vi "Run RT VI in project.vi"(5 "project target":string, 6 "configuration file path":path, 7 "ip address":string, 8 "error in (no error)":errorcluster, 9 "target alias":string, 10 "vi name":string, 11 "Project Path":path) -> (0 "error out":errorcluster, 1 "invoked VI error out":errorcluster, 2 "pass":bool, 3 "engine status":string)   [LabVIEW 2014]
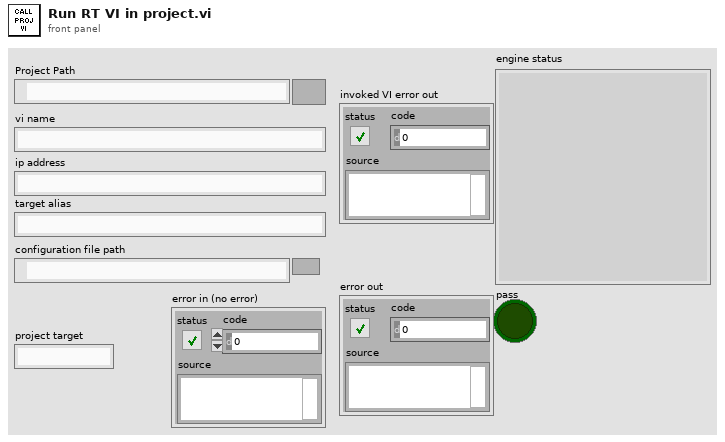
[diagram p1: front panel]
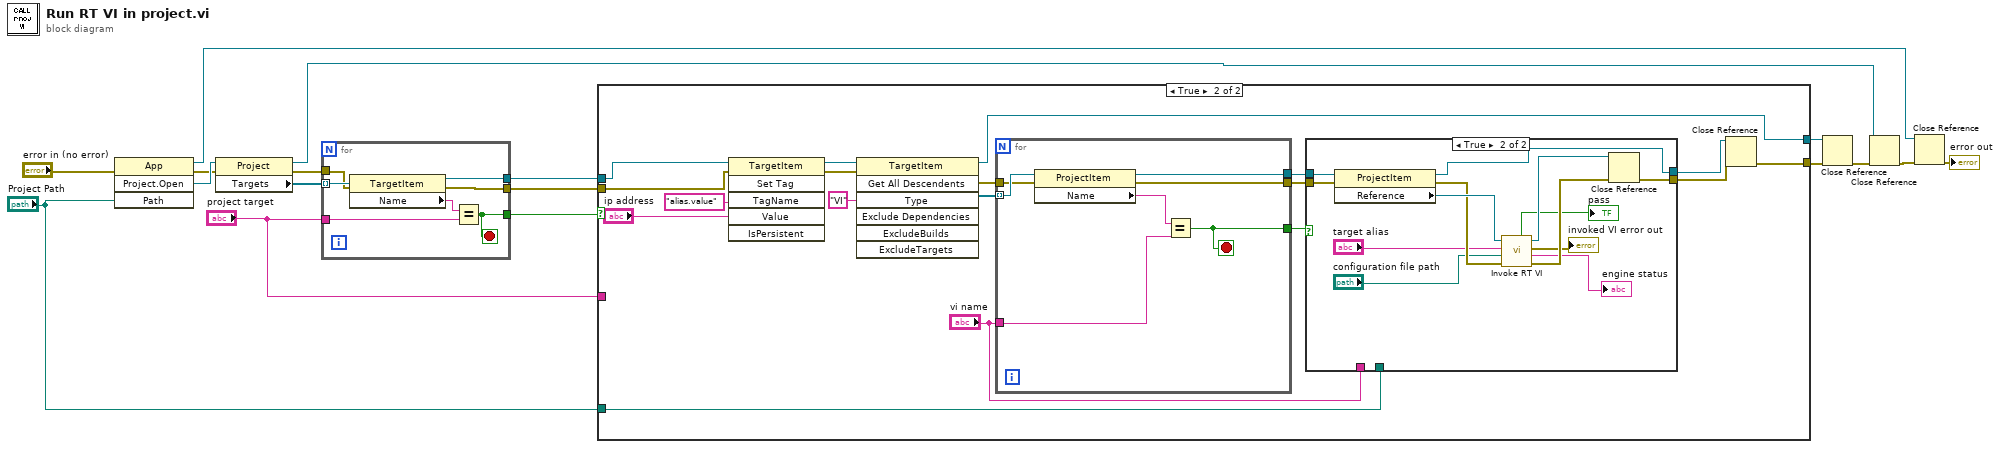
[diagram p0: block diagram]
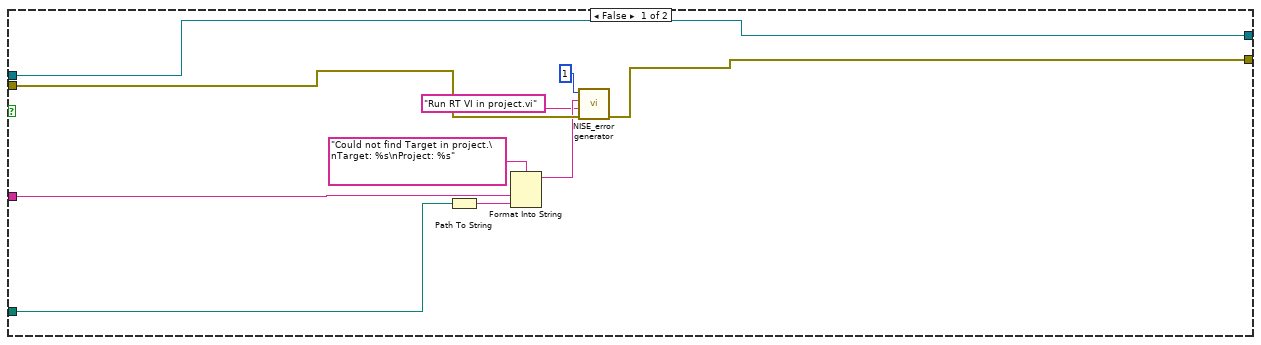
[diagram p2: hidden frame]
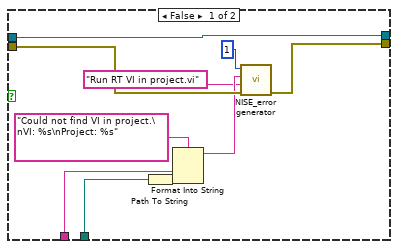
[diagram p3: hidden frame]
diagram:
  n1 = invoke class="App" method="Project.Open"(error in="error in (no error)", "Path"="Project Path") -> (reference out=w12:refnum<vi>, error out=w16:errorcluster, "Project:Open"=w17:refnum<vi>)  [unwired: 2 in, 1 out]
  n2 = property class="Project"(reference=w17, error in=w16) -> (reference out=w14:refnum<vi>, error out=w7:errorcluster, "Targets"=w15:refnum<vi>[])
  n3 = for {
    tunnel: w15 -> [w24] mode=indexing
    tunnel: [w23] -> w9
    tunnel: w7 -> [w21]
    tunnel: [w20] -> w6
    tunnel: [w19] -> w5
    tunnel: "project target" -> [w18]
    stop <- w19 stop-if-true
    n4 = property class="TargetItem"(reference=w24, error in=w21) -> (reference out=w23:refnum<vi>, error out=w20:errorcluster, "Name"=w22:string)
    n5 = Equal?(x=w22, y=w18) -> (x = y?=w19:bool)
  }
  n6 = case shown="True" w5 {
    tunnel: [w25 w35] -> w3
    tunnel: w9 -> [w34 w45]
    tunnel: "Project Path" -> [w33 w38]
    tunnel: w6 -> [w31 w37]
    tunnel: [w34 w36] -> w4
    tunnel: "project target" -> [w32 _]
    frame False {
      n7 = Path To String(path=w33) -> (string=w28:string)
      n8 = Format Into String(format string="Could not find Target in project.\nTarget: %s\nProject: %s" ("append error message"), w32, w28) -> (resulting string=w27:string)  [unwired: 2 in, 1 out]
      n9 = call <vilib>:"NISE_error generator.vi"("error in"=w31, "source"="Run RT VI in project.vi", "append error message"=w27, "error code (0)"=1) -> ("error out"=w25:errorcluster)  [unwired: 5 in]
    }
    frame True {
      n10 = invoke class="TargetItem" method="Set Tag"(reference=w45, error in=w37, "TagName"="alias.value" ("Tag Name"), "Value"="ip address") -> (reference out=w41:refnum<vi>, error out=w42:errorcluster)  [unwired: 2 in, 4 out]
      n11 = invoke class="TargetItem" method="Get All Descendents"(reference=w41, error in=w42, "Type"="VI") -> (reference out=w36:refnum<vi>, error out=w51:errorcluster, "All Descendents"=w52:refnum<vi>[])  [unwired: 4 in, 4 out]
      n12 = for {
        tunnel: w52 -> [w82] mode=indexing
        tunnel: w51 -> [w81]
        tunnel: "vi name" -> [w80]
        tunnel: [w79] -> w50
        tunnel: [w78] -> w49
        tunnel: [w77] -> w48
        stop <- w77 stop-if-true
        n13 = property class="ProjectItem"(reference=w82, error in=w81) -> (reference out=w79:refnum<vi>, error out=w78:errorcluster, "Name"=w76:string)
        n14 = Equal?(x=w76, y=w80) -> (x = y?=w77:bool)
      }
      n15 = case shown="True" w48 {
        tunnel: w50 -> [w62 w75]
        tunnel: w49 -> [w61 w74]
        tunnel: [w60 w73] -> w47
        tunnel: [w62 w72] -> w46
        tunnel: "vi name" -> [w57 _]
        tunnel: w38 -> [w56 _]
        frame False {
          n16 = Path To String(path=w56) -> (string=w55:string)
          n17 = Format Into String(format string="Could not find VI in project.\nVI: %s\nProject: %s" ("append error message"), w57, w55) -> (resulting string=w54:string)  [unwired: 2 in, 1 out]
          n18 = call <vilib>:"NISE_error generator.vi"("error in"=w61, "source"="Run RT VI in project.vi", "append error message"=w54, "error code (0)"=1) -> ("error out"=w60:errorcluster)  [unwired: 5 in]
        }
        frame True {
          n19 = property class="ProjectItem"(reference=w75, error in=w74) -> (reference out=w72:refnum<vi>, error out=w70:errorcluster, "Reference"=w71:refnum<vi>)
          n20 = call "Invoke RT VI.vi"("error in (no error)"=w70, "configuration file path"="configuration file path", "target alias"="target alias", "reference"=w71) -> ("error out"=w67:errorcluster, "engine status"=→"engine status":string, "invoked VI error out"=→"invoked VI error out":errorcluster, "reference out"=w66:refnum<vi>, "pass"=→"pass":bool)  [unwired: 3 in]
          n21 = Close Reference(reference=w66, error in (no error)=w67) -> (error out=w73:errorcluster)
        }
      }
      n22 = Close Reference(reference=w46, error in (no error)=w47) -> (error out=w35:errorcluster)
    }
  }
  n23 = Close Reference(reference=w4, error in (no error)=w3) -> (error out=w2:errorcluster)
  n24 = Close Reference(reference=w14, error in (no error)=w2) -> (error out=w13:errorcluster)
  n25 = Close Reference(reference=w12, error in (no error)=w13) -> (error out=→"error out":errorcluster)
